vi "Czas.vi"(7 "State":T1(ring), 8 "error in":errorcluster) -> (0 "error out":errorcluster, 1 "Time left":dbl, 2 "Elapsed Time":dbl, 3 "Time":bool, 5 "Pause":bool)   [LabVIEW 2020]
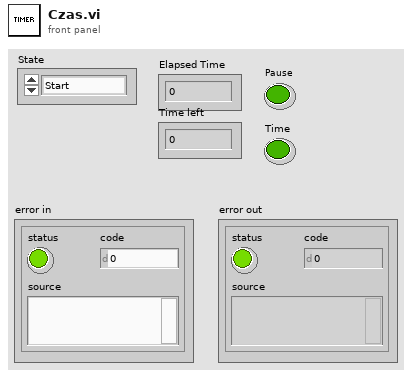
[diagram p1: front panel]
types:
  T1 = enum16{"Start", "Initialize", "Elapsed", "Pause"}
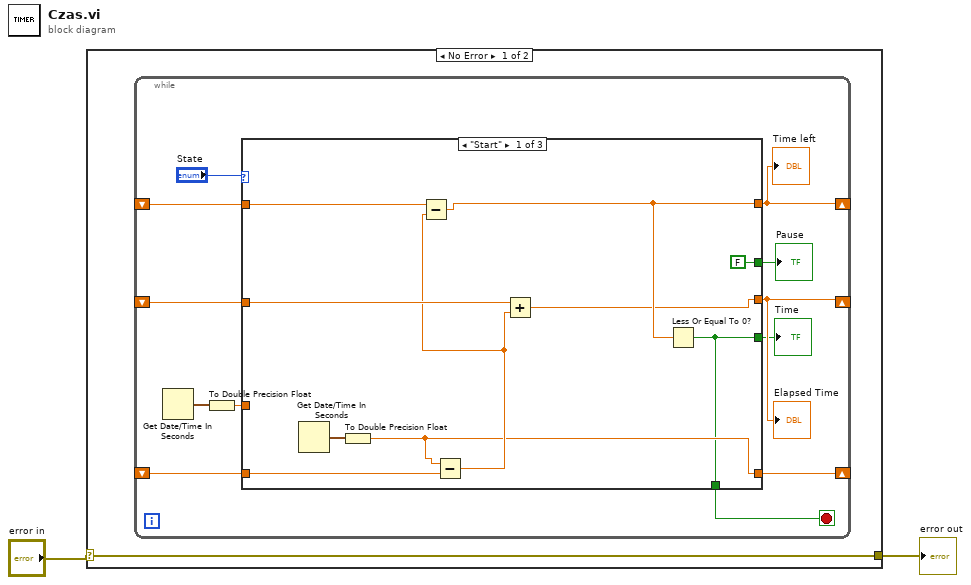
[diagram p0: block diagram]
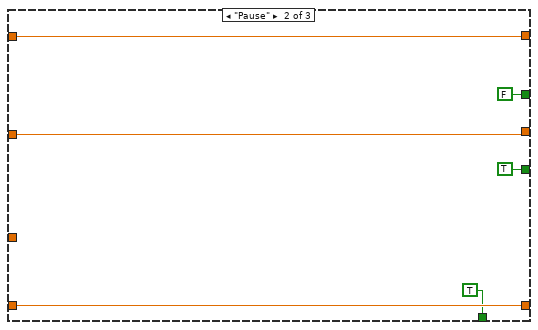
[diagram p2: hidden frame]
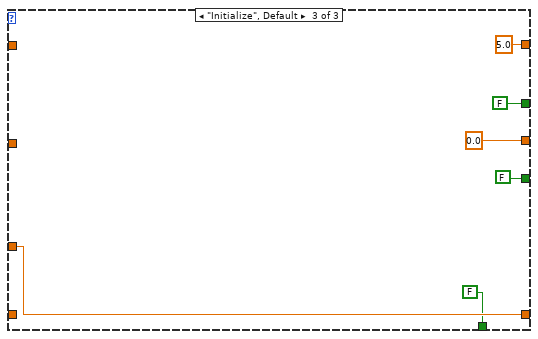
[diagram p3: hidden frame]
diagram:
  n1 = case shown="No Error" "error in" {
    selector: "error in" -> [w3 w38]
    tunnel: [w3 w38] -> w1
    frame No Error {
      n2 = while {
        shift-right: [w14] -> _
        shift-left: _ -> [w7]
        shift-right: [w13] -> _
        shift-left: _ -> [w6]
        shift-right: [w8] -> _
        shift-left: _ -> [w5]
        stop <- w4 stop-if-true
        n3 = Get Date/Time In Seconds() -> (seconds since 1Jan1904=w10:timestamp)
        n4 = To Double Precision Float(number=w10) -> (double precision float=w9:dbl)
        n5 = case shown="\"Start\"" "State" {
          tunnel: [w23 w31 5.0] -> w14
          tunnel: [w21 w28 0.0] -> w13
          tunnel: [FALSE ("Pause") FALSE ("Pause") FALSE ("Pause")] -> w12
          tunnel: [w16 TRUE ("Pause") FALSE ("Pause")] -> w11
          tunnel: w9 -> [_ _ w34]
          tunnel: [w18 w27 w34] -> w8
          tunnel: w7 -> [w24 w31 _]
          tunnel: w6 -> [w22 w28 _]
          tunnel: w5 -> [w20 w27 _]
          tunnel: [w16 TRUE FALSE] -> w4
          frame "Start" {
            n6 = Get Date/Time In Seconds() -> (seconds since 1Jan1904=w25:timestamp)
            n7 = To Double Precision Float(number=w25) -> (double precision float=w18:dbl)
            n8 = Subtract(x=w18, y=w20) -> (x-y=w19:dbl)
            n9 = Subtract(x=w24, y=w19) -> (x-y=w23:dbl)
            n10 = Add(x=w22, y=w19) -> (x+y=w21:dbl)
            n11 = Less Or Equal To 0?(x=w23) -> (x <= 0?=w16:bool)
          }
          frame "Pause" {
          }
          frame "Initialize", Default {
          }
        }
        "Pause" <- w12
        "Time" <- w11
        "Elapsed Time" <- w13
        "Time left" <- w14
      }
    }
    frame Error {
    }
  }
  "error out" <- w1
